vi "Protocol.Network.Command Handler.vi"(8 "error in (no error)":errorcluster, 11 "J1939 Main Configuration":T1 {"Stream Refs"."Port Settings"."FD ISO Mode" items=["ISO", "Non ISO", "ISO Legacy"]; "Stream Refs"."Port Settings"."Termination" items=["Off", "On"]; "Stream Refs"."Port Settings"."Mode" items=["CAN 2.0", "CAN FD", "CAN FD+BRS"]}) -> (0 "error out":errorcluster)   [LabVIEW 2023, in "J1939 Addon Engine.lvlib"]
uses:
  J1939 Addon Engine.lvlib
  Types/Protocol.Configuration.ctl
  <vilib>/NI/NI VeriStand Addon Network Comm/Engine/VeriStand Comm.lvclass
  <vilib>/NI/NIVS Inline Async API/_VS Inline Async API/Process/Process.lvclass
  Types/Protocol.Refs.ctl
  Support Libraries/J1939 Utilities/Types/CAN Outgoing Message Cluster.ctl
  Types/Protocol.RQST Lookup Table Reference.ctl
  Types/Protocol.Address Table Reference.ctl
  Types/Protocol.XNET Settings.ctl
  <vilib>/NI/NIVS Inline Async API/_Data Access Engine/Data Access Engine/Types/Read.DVR.ctl
  <vilib>/NI/NIVS Inline Async API/_Data Access Engine/Access Type Classes/Read/Read.lvclass
  <vilib>/NI/NIVS Inline Async API/_Data Access Engine/Data Access Engine/Types/Write.DVR.ctl
  <vilib>/NI/NIVS Inline Async API/_Data Access Engine/Access Type Classes/Write/Write.lvclass
  Types/CounterAndProtectionFrames.ctl
  SubModules/Frame-Protection-Support/Source/Engine/Types/RT Frame Settings.ctl
  SubModules/Frame-Protection-Support/Source/Shared/Types/Exported Frame Type.ctl
  SubModules/Frame-Protection-Support/Source/Engine/Types/RT Protection Configuration.ctl
  SubModules/Frame-Protection-Support/Source/Shared/Types/Protection Type.ctl
  SubModules/Frame-Protection-Support/Source/Shared/Types/XNET Signal Configuration.ctl
  SubModules/Frame-Protection-Support/Source/Shared/Types/Exported Counter Settings.ctl
  SubModules/Frame-Protection-Support/Source/Shared/Types/Exported Event Trigger Type.ctl
  SubModules/CAN-Streaming-Support/Source/Addon/Addon Engine/Types/Engine Stream Refs.ctl
  SubModules/CAN-Streaming-Support/Source/Addon/Addon Shared/Types/Direction Filter.ctl
  SubModules/CAN-Streaming-Support/Source/Addon/Addon Shared/Types/Type Filter.ctl
  SubModules/CAN-Streaming-Support/Source/Addon/Addon Shared/Types/Filter Parameters.ctl
  SubModules/CAN-Streaming-Support/Source/Addon/Addon Engine/Types/Engine Stream Port Settings.ctl
  <vilib>/NI/NI VeriStand Addon Network Comm/Engine/VeriStand Comm.lvclass/VeriStand Comm.ctl
  Addon Shared/Types/Request Message.ctl
  Types/Protocol.Address Lookup Table Action.ctl
  <vilib>/NI/NIVS Inline Async API/_VS Inline Async API/Process/Process.lvclass/Process.ctl
  Support Libraries/J1939 Utilities/SubVIs/Convert CAN Arb ID to J1939 ID.vi
  <vilib>/NI/NIVS Inline Async API/_VS Inline Async API/Error Handling Process/SubVIs/Error.ConvertArray.vi
  <vilib>/NI/AMC/Read Next Message.vi
  <vilib>/NI/Tools/Keyed Array/Index.vi
  Support Libraries/J1939 Utilities/Common Messages.vi
  Support Libraries/J1939 Utilities/SubVIs/Request.vi
  Protocol.RQST Lookup Table Act.vi
  <vilib>/NI/AMC/Send Local Message.vi
  <vilib>/NI/AMC/Read Termination Message.vi
  <vilib>/NI/Tools/Keyed Array/Map String.vi
  Support Libraries/J1939 Utilities/SubVIs/Convert J1939 ID to CAN Arb ID.vi
  <vilib>/NI/AMC/Create Single Message.vi
  <vilib>/NI/AMC/Update Message Routing Info.vi
  <vilib>/NI/Tools/String/Get Case Matching.vi
  <vilib>/NI/NI VeriStand Addon Network Comm/Shared/Comm Constants.vi
  <vilib>/NI/AMC/Globals.vi
  Protocol.RQST Lookup Table.vi
  <vilib>/xnet/xnet.llb/XNET Read (State CAN Comm).vi
  <vilib>/Utility/SystemLogging/Write to System Log.vi
  Protocol.Address Lookup Table.vi
  <vilib>/NI/AMC/Send Message.vi
  Addon Shared/J1939 Addon Shared.lvlib
  Support Libraries/J1939 Utilities/J1939 Utilities.lvlib
  SubModules/CAN-Streaming-Support/Source/Addon/Addon Engine/CAN Stream Support Engine.lvlib
  SubModules/CAN-Streaming-Support/Source/Addon/Addon Shared/CAN Stream Support Shared.lvlib
  <vilib>/NI/NIVS Inline Async API/_Data Access Engine/Data Access Engine/Data Access Engine.lvclass
  SubModules/Frame-Protection-Support/Source/Engine/Protection and Counter Support Engine.lvlib
  SubModules/Frame-Protection-Support/Source/Shared/Protection and Counter Support Shared.lvlib
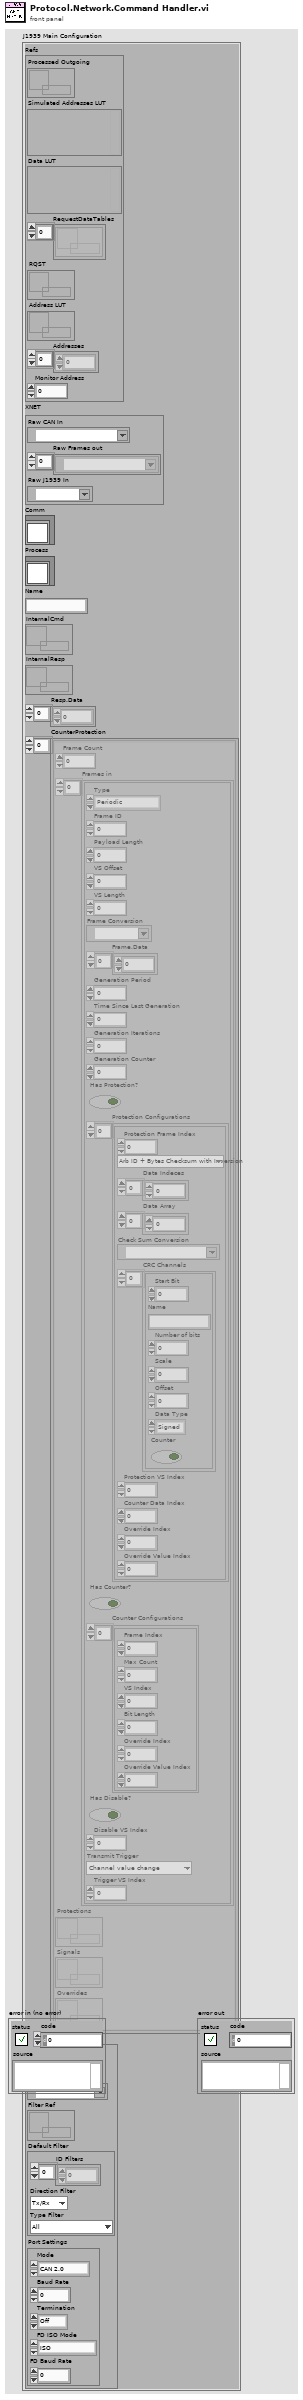
[diagram p1: front panel]
types:
  T1 = typedef "J1939 Addon Engine.lvlib/Protocol.Configuration.ctl" = cluster{"Refs":T2, "XNET":T5, "Comm":refnum<class "VeriStand Comm.lvclass">, "Process":refnum<class "Process.lvclass">, "Name":string, "InternalCmd":T6, "InternalResp":T7, "Resp.Data":dbl[], "CounterProtection":T8[], "Stream Refs":T16}
  T2 = typedef "J1939 Addon Engine.lvlib/Protocol.Refs.ctl" = cluster{"Processed Outgoing":refnum<queue>, "Simulated Addresses LUT":variant, "Data LUT":variant, "RequestDataTables":refnum<k33>[], "RQST":T3, "Address LUT":T4, "Addresses":u8[], "Monitor Address":u8}
  T3 = typedef "J1939 Addon Engine.lvlib/Protocol.RQST Lookup Table Reference.ctl" = refnum<data-value>
  T4 = typedef "J1939 Addon Engine.lvlib/Protocol.Address Table Reference.ctl" = refnum<data-value>
  T5 = typedef "J1939 Addon Engine.lvlib/Protocol.XNET Settings.ctl" = cluster{"Raw CAN In":refnum<k21>, "Raw Frames out":refnum<k21>[], "Raw J1939 In":refnum<k21>}
  T6 = typedef "Data Access Engine.lvlib/Data Access Engine.lvclass/Read.DVR.ctl" = refnum<data-value>
  T7 = typedef "Data Access Engine.lvlib/Data Access Engine.lvclass/Write.DVR.ctl" = refnum<data-value>
  T8 = typedef "J1939 Addon Engine.lvlib/CounterAndProtectionFrames.ctl" = cluster{"Frame Count":i32, "Frames in":T9[], "Protections":T7, "Signals":T6, "Overrides":T6}
  T9 = typedef "Protection and Counter Support Engine.lvlib/RT Frame Settings.ctl" = cluster{"Type":T10, "Frame ID":u32, "Payload Length":u32, "VS Offset":i32, "VS Length":i32, "Frame Conversion":refnum<k21>, "Frame.Data":dbl[], "Generation Period":u32, "Time Since Last Generation":u32, "Generation Iterations":u32, "Generation Counter":u32, "Has Protection?":bool, "Protection Configurations":T11[], "Has Counter?":bool, "Counter Configurations":T14[], "Has Disable?":bool, "Disable VS Index":i32, "Transmit Trigger":T15, "Trigger VS Index":i32}
  T10 = typedef "Protection and Counter Support Shared.lvlib/Exported Frame Type.ctl" = enum16{"Periodic", "Event", "Periodic/Event"}
  T11 = typedef "Protection and Counter Support Engine.lvlib/RT Protection Configuration.ctl" = cluster{"Protection Frame Index":i32, "Protection Type":T12, "Data Indeces":i32[], "Data Array":dbl[], "Check Sum Conversion":refnum<k21>, "CRC Channels":T13[], "Protection VS Index":i32, "Counter Data Index":i32, "Override Index":i32, "Override Value Index":i32}
  T12 = typedef "Protection and Counter Support Shared.lvlib/Protection Type.ctl" = enum16{"Arb ID + Bytes Checksum with Inversion", "Arb ID + Bytes CRC with Inversion", "Reversed Raw Signal Checksum with Inversion", "Concatenated Two's Compliment"}
  T13 = typedef "Protection and Counter Support Shared.lvlib/XNET Signal Configuration.ctl" = cluster{"Start Bit":i32, "Name":string, "Number of bits":i32, "Scale":dbl, "Offset":dbl, "Data Type":u32, "Counter":bool}
  T14 = typedef "Protection and Counter Support Shared.lvlib/Exported Counter Settings.ctl" = cluster{"Frame Index":i32, "Max Count":dbl, "VS Index":i32, "Bit Length":i64, "Override Index":i32, "Override Value Index":i32}
  T15 = typedef "Protection and Counter Support Shared.lvlib/Exported Event Trigger Type.ctl" = enum16{"Channel value change", "Trigger channel (not zero)", "Channel value change or trigger channel (not zero)", "Trigger channel (any value change)", "Channel value change or trigger channel (any value change)"}
  T16 = typedef "CAN Stream Support Engine.lvlib/Engine Stream Refs.ctl" = cluster{"Addon":string, "Port":refnum<k21>, "Filter Ref":refnum<data-value>, "Default Filter":T17, "Port Settings":T20}
  T17 = typedef "CAN Stream Support Shared.lvlib/Filter Parameters.ctl" = cluster{"ID Filters":u32[], "Direction Filter":T18, "Type Filter":T19}
  T18 = typedef "CAN Stream Support Shared.lvlib/Direction Filter.ctl" = enum16{"Tx/Rx", "Rx", "Tx"}
  T19 = typedef "CAN Stream Support Shared.lvlib/Type Filter.ctl" = enum16{"All", "CAN Data", "CAN Remote", "CAN Bus Error", "CAN 2.0 Data", "CAN FD Data", "CAN FD+BRS Data", "J1939 Data", "Delay", "Log Trigger", "Start Trigger"}
  T20 = typedef "CAN Stream Support Engine.lvlib/Engine Stream Port Settings.ctl" = cluster{"Mode":u32, "Baud Rate":u64, "Termination":u32, "FD ISO Mode":u32, "FD Baud Rate":u64}
  T21 = typedef "J1939 Addon Shared.lvlib/Request Message.ctl" = cluster{"PGN":u32, "DA":u8, "Ignore Response":bool}
  T22 = typedef "J1939 Utilities.lvlib/CAN Outgoing Message Cluster.ctl" = cluster{"Identifier":u32, "Data":u8[]}
  T23 = typedef "J1939 Addon Engine.lvlib/Protocol.Address Lookup Table Action.ctl" = enum16{"Initialize", "Add", "Get", "Remove", "Get All"}
  T24 = typedef "NI VeriStand Addon Network Comm.lvlib/VeriStand Comm.lvclass/Response Information.ctl" = cluster{"response name":string, "responseQ":string}
  T25 = typedef "XNET Frame CAN.ctl" = cluster{"timestamp":timestamp, "payload":u8[], "identifier":u32, "type":T26, "extended?":bool, "echo?":bool}
  T26 = typedef "XNET Frame Type CAN.ctl" = u8
  T27 = cluster{"ID Filters":u32[], "Direction Filter":T18, "Type Filter":T19}
  T28 = typedef "XNET CAN Comm.ctl" = cluster{"fault code":i32, "fault?":bool, "communication state":T29, "last error":T30, "receive error counter":u8, "transmit error counter":u8, "transceiver error?":bool, "sleep?":bool}
  T29 = typedef "XNET CAN Comm State.ctl" = u8
  T30 = typedef "XNET CAN Last Err.ctl" = u8
  T31 = typedef "J1939 Addon Shared.lvlib/Address Lookup Table Data.ctl" = cluster{"Name":u8[], "Address":u8}
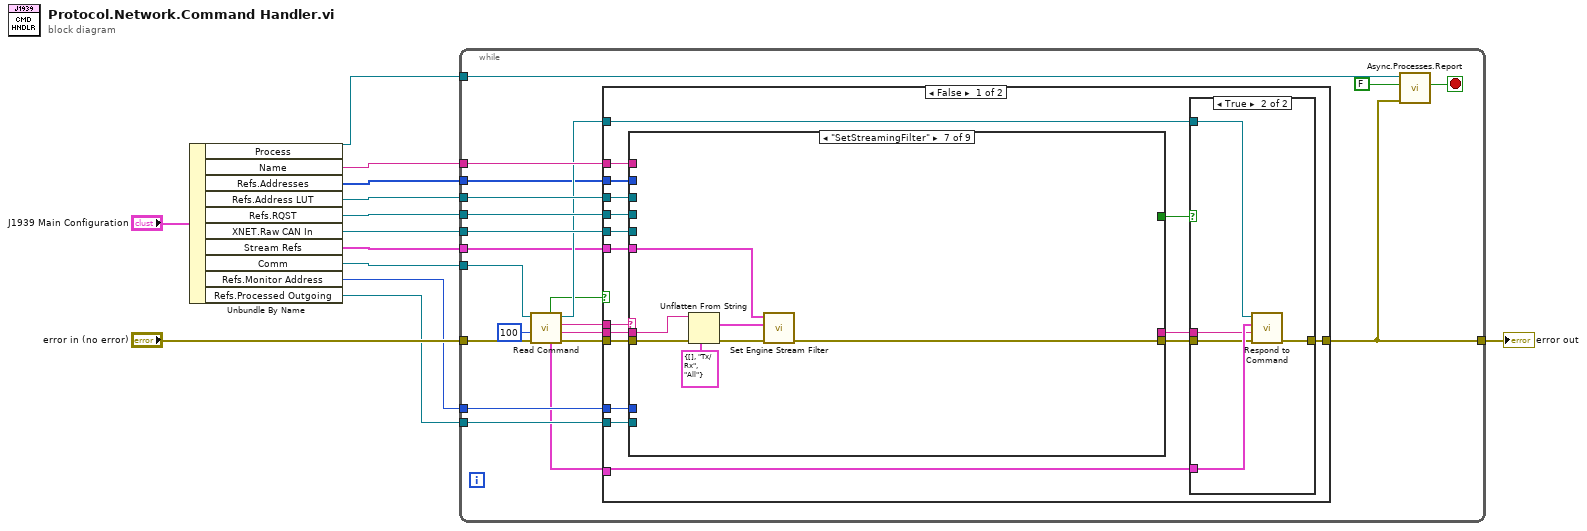
[diagram p0: block diagram]
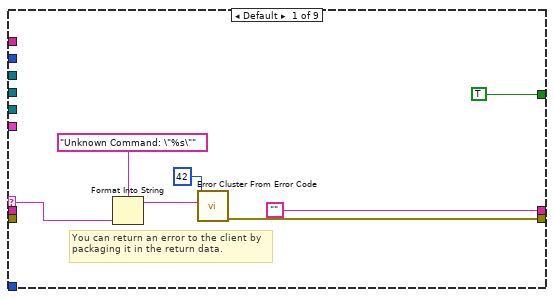
[diagram p3: hidden frame]
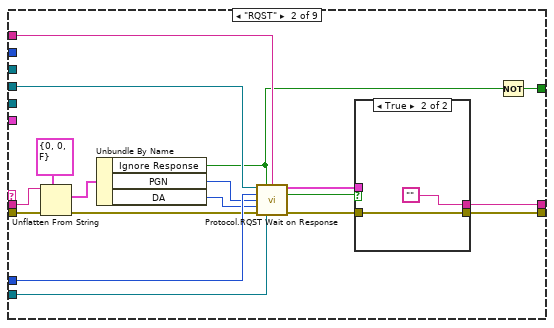
[diagram p4: hidden frame]
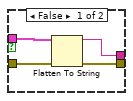
[diagram p5: hidden frame]
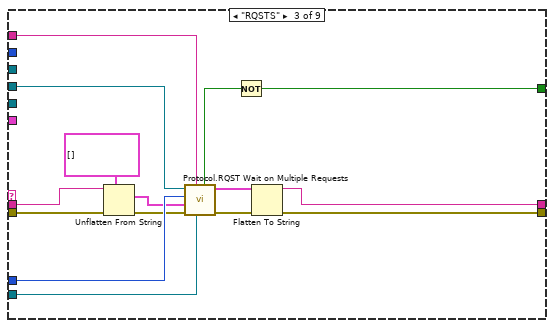
[diagram p6: hidden frame]
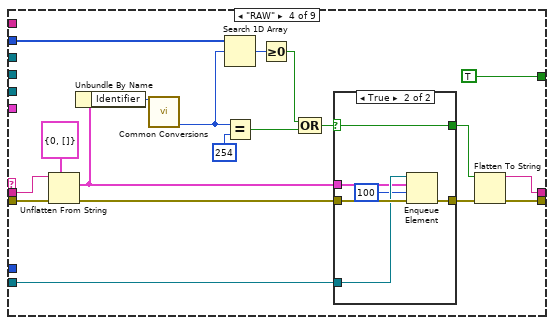
[diagram p7: hidden frame]
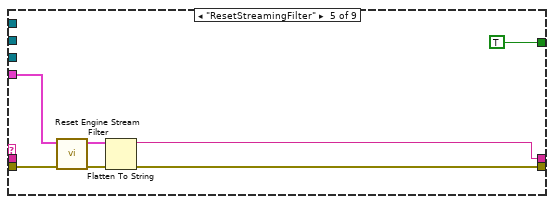
[diagram p9: hidden frame]
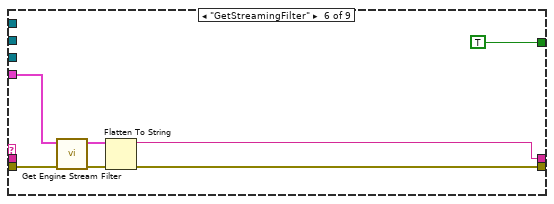
[diagram p10: hidden frame]
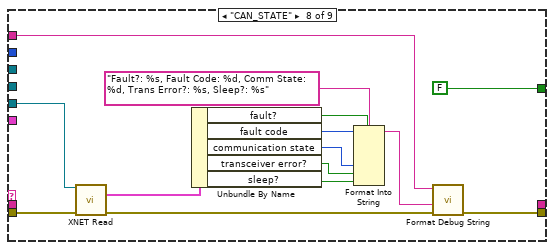
[diagram p11: hidden frame]
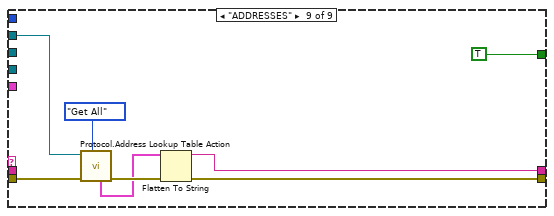
[diagram p12: hidden frame]
diagram:
  n1 = Unbundle By Name("J1939 Main Configuration") -> ("Process"=w4:refnum<class "Process.lvclass">, "Name"=w5:string, "Refs.Addresses"=w2:u8[], "Refs.Address LUT"=w6:T4, "Refs.RQST"=w7:T3, "XNET.Raw CAN In"=w8:refnum<k21>, "Stream Refs"=w1:T16, "Comm"=w9:refnum<class "VeriStand Comm.lvclass">, "Refs.Monitor Address"=w10:u8, "Refs.Processed Outgoing"=w11:refnum<queue>)
  n2 = while {
    tunnel: "error in (no error)" -> [w31]
    tunnel: [w23] -> w12
    tunnel: w4 -> [w33]
    tunnel: w9 -> [w30]
    tunnel: w5 -> [w29]
    tunnel: w8 -> [w28]
    tunnel: w11 -> [w27]
    tunnel: w10 -> [w26]
    tunnel: w7 -> [w25]
    tunnel: w6 -> [w24]
    tunnel: w2 -> [w15]
    tunnel: w1 -> [w14]
    stop <- w34 stop-if-true
    n3 = call <vilib>:"Read Command.vi"("error in (no error)"=w31, "timeout (100 ms)"=100, "VeriStand Comm in"=w30) -> ("error out"=w21:errorcluster, "message value"=w19:string, "message name"=w20:string, "VeriStand Comm out"=w17:refnum<class "VeriStand Comm.lvclass">, "ResponseInfo"=w18:T24, "timed out?"=w16:bool)  [unwired: 3 in]
    n4 = case shown="False" w16 {
      tunnel: w29 -> [w51 _]
      tunnel: w28 -> [w50 _]
      tunnel: w27 -> [w49 _]
      tunnel: w26 -> [w48 _]
      tunnel: w25 -> [w47 _]
      tunnel: w24 -> [w46 _]
      tunnel: [w45 w174] -> w23
      tunnel: w21 -> [w44 w174]
      tunnel: w20 -> [w43 _]
      tunnel: w19 -> [w42 _]
      tunnel: w18 -> [w41 _]
      tunnel: w17 -> [w40 _]
      tunnel: w15 -> [w36 _]
      tunnel: w14 -> [w35 _]
      frame False {
        n5 = case shown="\"SetStreamingFilter\"" w43 {
          selector: w43 -> [w60 _ _ _ _ _ _ _ _]
          tunnel: w42 -> [_ w69 w89 w121 _ _ w147 _ _]
          tunnel: [w61 w81 w90 w105 w133 w140 w150 w152 w167] -> w38
          tunnel: ["" ("data string") w78 w103 w104 w132 w139 _ _ w168] -> w39
          tunnel: w49 -> [_ w76 w101 w119 _ _ _ _ _]
          tunnel: w44 -> [_ w75 w93 w122 w134 w141 w149 w165 w172]
          tunnel: w47 -> [_ w68 w100 _ _ _ _ _ _]
          tunnel: w48 -> [_ w82 w99 _ _ _ _ _ _]
          tunnel: w46 -> [_ _ _ _ _ _ _ _ w171]
          tunnel: w51 -> [_ w67 w96 _ _ _ _ w155 _]
          tunnel: w50 -> [_ _ _ _ _ _ _ w164 _]
          tunnel: [TRUE w65 w94 TRUE TRUE TRUE _ FALSE TRUE] -> w37
          tunnel: w36 -> [_ _ _ w114 _ _ _ _ _]
          tunnel: w35 -> [_ _ _ _ w137 w144 w151 _ _]
          frame Default {
            # "You can return an error to the client by packaging it in the return data."
            n6 = Format Into String(format string="Unknown Command: \"%s\"", w60) -> (resulting string=w62:string)  [unwired: 2 in, 1 out]
            n7 = call <vilib>:"Error Cluster From Error Code.vi"("error message (\"\")"=w62, "error code (0)"=42) -> ("error out"=w61:errorcluster)  [unwired: 7 in]
          }
          frame "RQST" {
            n8 = Unflatten From String(type=T21 {"PGN"=0, "DA"=0, "Ignore Response"=FALSE} ("Cluster"), binary string=w69, error in (no error)=w75) -> (value=w72:T21, error out=w74:errorcluster)  [unwired: 2 in, 1 out]
            n9 = Unbundle By Name(w72) -> ("Ignore Response"=w66:bool, "PGN"=w71:u32, "DA"=w70:u8)
            n10 = call "Protocol.RQST Wait on Response.vi"("ref in"=w68, "Ignore Response"=w66, "Name"=w67, "Source Address"=w82, "PGN"=w71, "DA"=w70, "error in (no error)"=w74, "Processed Outgoing"=w76) -> ("element"=w77:T25, "timed out?"=w79:bool, "error out"=w80:errorcluster)  [unwired: 4 in, 1 out]
            n11 = case shown="True" w79 {
              tunnel: [w84 w88] -> w81
              tunnel: w80 -> [w85 w88]
              tunnel: [w83 ""] -> w78
              tunnel: w77 -> [w86 _]
              frame False {
                n12 = Flatten To String(anything=w86, error in (no error)=w85) -> (data string=w83:string, error out=w84:errorcluster)  [unwired: 2 in, 1 out]
              }
              frame True {
              }
            }
            n13 = Not(x=w66) -> (.not. x?=w65:bool)
          }
          frame "RQSTS" {
            n14 = Unflatten From String(type=T21[] [], binary string=w89, error in (no error)=w93) -> (value=w98:T21[], error out=w92:errorcluster)  [unwired: 2 in, 1 out]
            n15 = call "Protocol.RQST Wait on Multiple Requests.vi"("Processed Outgoing"=w101, "Name"=w96, "error in (no error)"=w92, "value"=w98, "Source Address"=w99, "ref in"=w100) -> ("error out"=w91:errorcluster, "Elements"=w97:T25[], "Ignore Response?"=w95:bool)  [unwired: 1 in, 2 out]
            n16 = Not(x=w95) -> (.not. x?=w94:bool)
            n17 = Flatten To String(anything=w97, error in (no error)=w91) -> (data string=w103:string, error out=w90:errorcluster)  [unwired: 2 in, 1 out]
          }
          frame "RAW" {
            n18 = Unflatten From String(type=T22 {"Identifier"=0, "Data"=[]} ("Data to Send"), binary string=w121, error in (no error)=w122) -> (value=w117:T22, error out=w108:errorcluster)  [unwired: 2 in, 1 out]
            n19 = Unbundle By Name(w117) -> ("Identifier"=w116:u32)
            n20 = call-poly "Common Conversions.vi"("Arb ID"=w116) -> ("Source Address"=w113:u8)  [unwired: 11 in, 3 out]
            n21 = Search 1D Array(1D array=w114, element=w113) -> (index of element=w112:i32)  [unwired: 1 in]
            n22 = Equal?(x=w113, y=u8 254) -> (x = y?=w110:bool)
            n23 = Greater Or Equal To 0?(x=w112) -> (x >= 0?=w111:bool)
            n24 = Compound Arithmetic op=OR(w111, w110) -> (w109:bool)
            n25 = case shown="True" w109 {
              selector: w109 -> [w123 w125]
              tunnel: w108 -> [w124 w130]
              tunnel: w119 -> [_ w129]
              tunnel: [w124 w127] -> w106
              tunnel: w117 -> [_ w126]
              tunnel: [w123 w125] -> w107
              frame False {
              }
              frame True {
                n26 = Enqueue Element(queue=w129, element=w126, timeout in ms (-1)=100, error in (no error)=w130) -> (error out=w127:errorcluster)  [unwired: 2 out]
              }
            }
            n27 = Flatten To String(anything=w107, error in (no error)=w106) -> (data string=w104:string, error out=w105:errorcluster)  [unwired: 2 in, 1 out]
          }
          frame "ResetStreamingFilter" {
            n28 = call "Reset Engine Stream Filter.vi"("error in (no error)"=w134, "Refs"=w137) -> ("error out"=w135:errorcluster, "Filter"=w136:T17)  [unwired: 8 in]
            n29 = Flatten To String(anything=w136, error in (no error)=w135) -> (data string=w132:string, error out=w133:errorcluster)  [unwired: 2 in, 1 out]
          }
          frame "GetStreamingFilter" {
            n30 = call "Get Engine Stream Filter.vi"("error in (no error)"=w141, "Refs"=w144) -> ("error out"=w142:errorcluster, "Filter"=w143:T27)  [unwired: 8 in]
            n31 = Flatten To String(anything=w143, error in (no error)=w142) -> (data string=w139:string, error out=w140:errorcluster)  [unwired: 2 in, 1 out]
          }
          frame "SetStreamingFilter" {
            n32 = Unflatten From String(type=T17 {"ID Filters"=[], "Direction Filter"=enum."Tx/Rx", "Type Filter"=enum."All"} ("Filter"), binary string=w147, error in (no error)=w149) -> (value=w145:T17, error out=w148:errorcluster)  [unwired: 2 in, 1 out]
            n33 = call "Set Engine Stream Filter.vi"("error in (no error)"=w148, "Filter"=w145, "Refs"=w151) -> ("error out"=w150:errorcluster)  [unwired: 8 in]
          }
          frame "CAN_STATE" {
            n34 = call-poly <vilib>:"XNET Read.vi"("session in"=w164, "error in (no error)"=w165) -> ("CAN comm"=w163:T28, "error out"=w153:errorcluster)  [unwired: 11 in, 1 out]
            n35 = Unbundle By Name(w163) -> ("fault?"=w162:bool, "fault code"=w161:i32, "communication state"=w160:T29, "transceiver error?"=w159:bool, "sleep?"=w158:bool)
            n36 = Format Into String(format string="Fault?: %s, Fault Code: %d, Comm State: %d, Trans Error?: %s, Sleep?: %s", w162, w161, w160, w159, w158) -> (resulting string=w154:string)  [unwired: 2 in, 1 out]
            n37 = call "Format Debug String.vi"("error in (no error)"=w153, "State"=w154, "Name"=w155) -> ("error out"=w152:errorcluster)  [unwired: 8 in]
          }
          frame "ADDRESSES" {
            n38 = call "Protocol.Address Lookup Table Action.vi"("Action"=Protocol.Address_Lookup_Table_Action."Get All", "error in (no error)"=w172, "ref in"=w171) -> ("error out"=w170:errorcluster, "All Data"=w169:T31[])  [unwired: 5 in, 2 out]
            n39 = Flatten To String(anything=w169, error in (no error)=w170) -> (data string=w168:string, error out=w167:errorcluster)  [unwired: 2 in, 1 out]
          }
        }
        n40 = case shown="True" w37 {
          tunnel: [w52 w57] -> w45
          tunnel: w41 -> [_ w56]
          tunnel: w40 -> [_ w55]
          tunnel: w39 -> [_ w54]
          tunnel: w38 -> [w52 w53]
          frame False {
          }
          frame True {
            n41 = call <vilib>:"Respond to Command.vi"("error in (no error)"=w53, "message value"=w54, "ResponseInfo"=w56, "VeriStand Comm in"=w55) -> ("error out"=w57:errorcluster)  [unwired: 5 in, 2 out]
          }
        }
      }
      frame True {
      }
    }
    n42 = call <vilib>:"Async.Processes.Report.vi"("Error"=w23, "Stop Async on Error?"=FALSE ("Stop on Error?"), "Process in"=w33) -> ("Stop"=w34:bool)  [unwired: 7 in, 1 out]
  }
  "error out" <- w12
